vi "StringPluckSim.vi"(6 "fretPos":dbl, 7 "offset":dbl, 8 "Initial Random Array":dbl[](array[numeric]), 9 "A":i32, 10 "Fs":i32, 11 "InitialArray":dbl[](array[numeric])) -> (3 "PluckedStringOut":dbl[](array[numeric]))   [LabVIEW 2016]
uses:
  <vilib>/Analysis/3filter.llb/IIR Filter (DBL).vi
  <vilib>/express/express arith-compare/Formula/XNode/ExpressFormulaBlockNode.xnode
  <vilib>/Analysis/NI_AALBase.lvlib
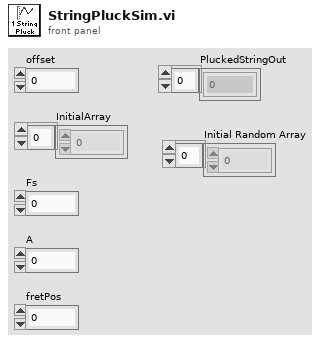
[diagram p1: front panel]
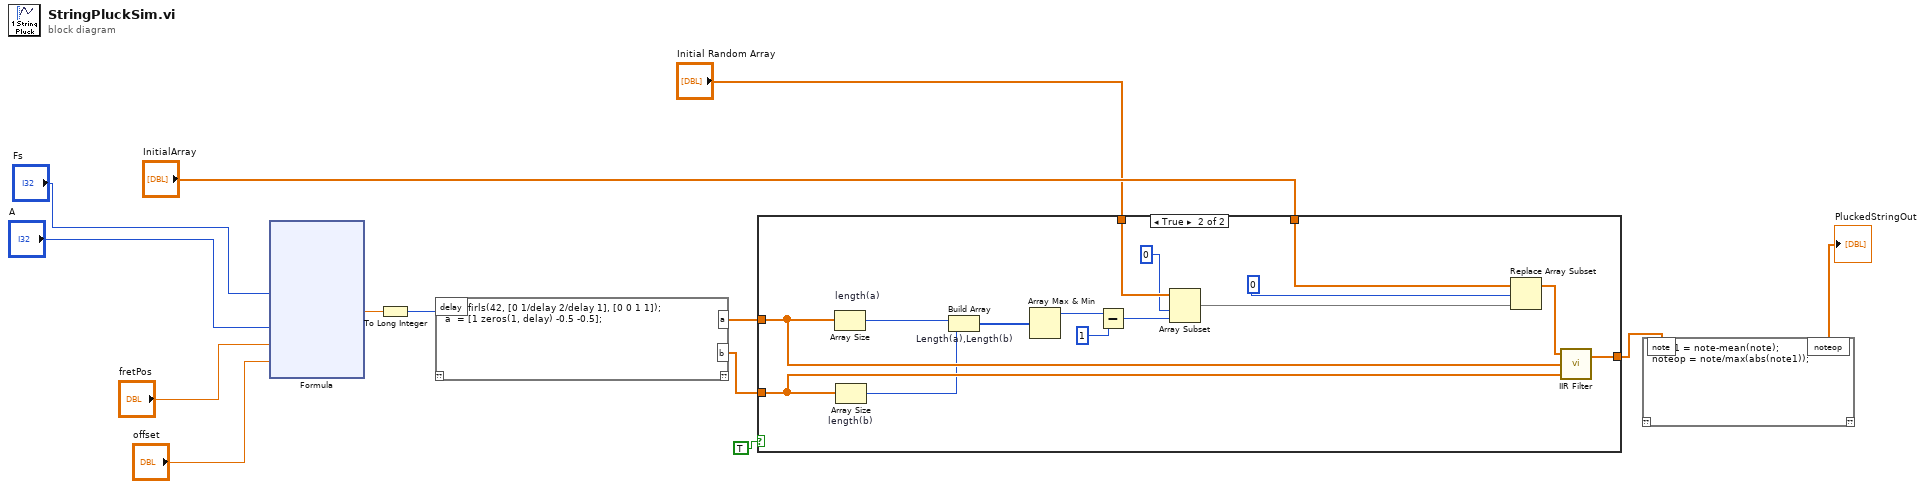
[diagram p0: block diagram]
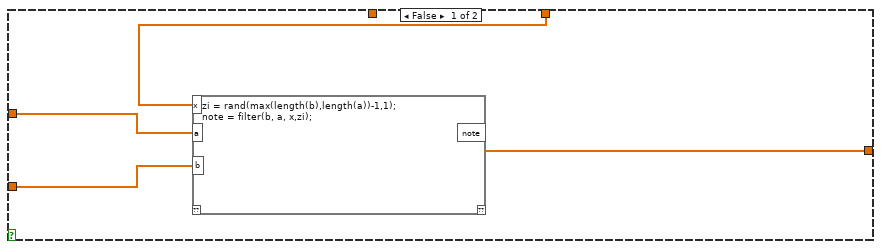
[diagram p2: hidden frame]
diagram:
  n1 = xnode "Formula"("SampleRate"="Fs", "A2"="A", "fretPos"="fretPos", "offset"="offset") -> ("Result"=w9:dbl)  [unwired: 1 in, 1 out]
  n2 = To Long Integer(number=w9) -> (32bit integer=w4:i32)
  n3 = script code="b  = firls(42, [0 1/delay 2/delay 1], [0 0 1 1]);\na  = [1 zeros(1, delay) -0.5 -0.5];"("delay"=w4) -> ("a"=w6:dbl[], "b"=w5:dbl[])  [unwired: 1 in, 1 out]
  n4 = case shown="True" TRUE {
    tunnel: [w14 w32] -> w8
    tunnel: "InitialArray" -> [w17 w31]
    tunnel: w6 -> [w16 w30]
    tunnel: w5 -> [w15 w29]
    tunnel: "Initial Random Array" -> [_ w20]
    frame False {
      n5 = script code="zi = rand(max(length(b),length(a))-1,1);\nnote = filter(b, a, x,zi);"("x"=w17, "a"=w16, "b"=w15) -> ("note"=w14:dbl[])  [unwired: 1 in, 1 out]
    }
    frame True {
      n6 = Array Size "length(a)"(array=w30) -> (size(s)=w22:i32)
      n7 = Array Size "length(b)"(array=w29) -> (size(s)=w23:i32)
      n8 = Build Array "Length(a),Length(b)"(w22, w23) -> (w24:i32[])
      n9 = Array Max & Min(array=w24) -> (max value=w25:i32)  [unwired: 3 out]
      n10 = Subtract(x=w25, y=1) -> (x-y=w21:i32)
      n11 = Array Subset(array=w20, index=0, length=w21) -> (w19:dbl[])
      n12 = Replace Array Subset(array=w31, new element=w19, index=0) -> (w28:dbl[])
      n13 = call-poly <vilib>:"IIR Filter.vi"("Forward Coefficients"=w29, "Reverse Coefficients"=w30, "X"=w28) -> ("Filtered X"=w32:dbl[])  [unwired: 1 in, 1 out]
    }
  }
  n14 = script code="note1 = note-mean(note);\nnoteop = note/max(abs(note1));"("note"=w8) -> ("noteop"=→"PluckedStringOut":dbl[])  [unwired: 1 in, 1 out]
